vi "Light cycling.vi"(0 "Base lights hold time":dbl=20.0 caption="Time Target (s)", 1 "rate pf change Base":dbl=20.0 format="%#_13g", 2 "rate pf change Lift":dbl=1.0 format="%#_13g") -> ()   [LabVIEW 2014]
uses:
  <vilib>/Rock Robotics/WPI/DriverStation/WPI_DriverStationAllianceInfo.ctl
  Robot Values.vi
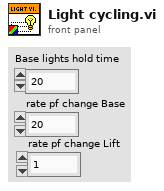
[diagram p1: front panel]
types:
  T1 = typedef "WPI_DriverStationAllianceInfo.ctl" = enum16{"Red", "Blue", "Invalid"}
  T2 = cluster{"Light level Base":dbl[], "Light level Lift":dbl[], "Light Level License plates":dbl[]}
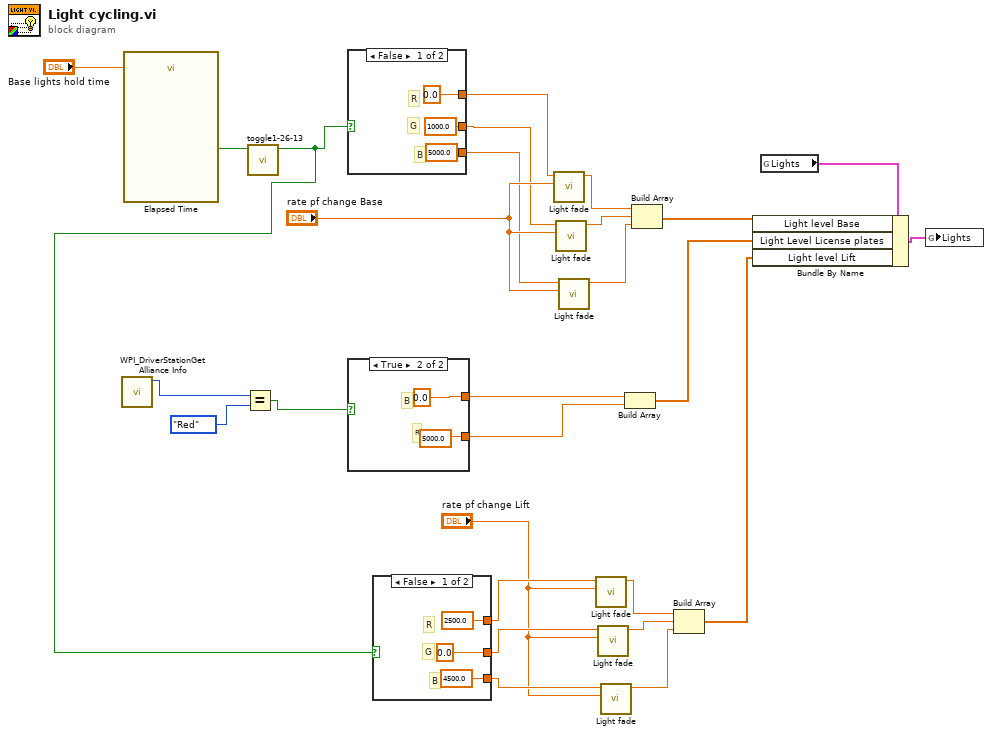
[diagram p0: block diagram]
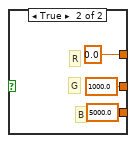
[diagram p2: hidden frame]
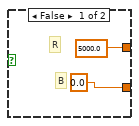
[diagram p3: hidden frame]
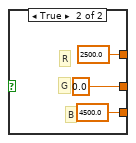
[diagram p4: hidden frame]
diagram:
  n1 = call <vilib>:"WPI_DriverStationGet Alliance Info.vi"() -> ("Alliance"=w14:T1)  [unwired: 10 in, 1 out]
  n2 = call "Elapsed Time"("Time Target (s)"="Base lights hold time") -> ("Time has Elapsed"=w27:bool)  [unwired: 11 in, 7 out]
  n3 = Equal?(x=w14, y=WPI_DriverStationAllianceInfo."Red") -> (x = y?=w12:bool)
  n4 = call "toggle1-26-13.vi"("input"=w27) -> ("output"=w1:bool)  [unwired: 10 in]
  n5 = case shown="False" w1 {
    tunnel: [0.0 2500.0] -> w25
    tunnel: [1000.0 0.0] -> w24
    tunnel: [5000.0 4500.0] -> w23
    frame False {
      # "B"
      # "G"
      # "R"
    }
    frame True {
      # "B"
      # "G"
      # "R"
    }
  }
  n6 = case shown="True" w12 {
    tunnel: [5000.0 0.0] -> w11
    tunnel: [0.0 5000.0] -> w10
    frame False {
      # "R"
      # "B"
    }
    frame True {
      # "R"
      # "B"
    }
  }
  n7 = case shown="False" w1 {
    tunnel: [2500.0 0.0] -> w5
    tunnel: [0.0 1000.0] -> w4
    tunnel: [4500.0 5000.0] -> w3
    frame False {
      # "B"
      # "G"
      # "R"
    }
    frame True {
      # "B"
      # "G"
      # "R"
    }
  }
  n8 = call "Light fade.vi"("rate pf change"="rate pf change Base", "value"=w25) -> ("Output"=w19:dbl)  [unwired: 9 in]
  n9 = call "Light fade.vi"("rate pf change"="rate pf change Base", "value"=w24) -> ("Output"=w18:dbl)  [unwired: 9 in]
  n10 = call "Light fade.vi"("rate pf change"="rate pf change Base", "value"=w23) -> ("Output"=w17:dbl)  [unwired: 9 in]
  n11 = call "Light fade.vi"("rate pf change"="rate pf change Lift", "value"=w5) -> ("Output"=w9:dbl)  [unwired: 9 in]
  n12 = call "Light fade.vi"("rate pf change"="rate pf change Lift", "value"=w4) -> ("Output"=w8:dbl)  [unwired: 9 in]
  n13 = call "Light fade.vi"("rate pf change"="rate pf change Lift", "value"=w3) -> ("Output"=w7:dbl)  [unwired: 9 in]
  n14 = Build Array(w11, w10) -> (w13:dbl[])
  n15 = Build Array(w19, w18, w17) -> (w20:dbl[])
  n16 = Build Array(w9, w8, w7) -> (w6:dbl[])
  n17 = global read "Robot Values.vi" "Lights"() -> (w21:T2)
  n18 = Bundle By Name(cluster=w21, "Light level Base"=w20, "Light Level License plates"=w13, "Light level Lift"=w6) -> (w22:T2)
  n19 = global write "Robot Values.vi" "Lights"(w22) -> ()
